vi "Power Spectrum.vi"   [LabVIEW 2024, in "NI_AALPro.lvlib"]
doc: "<p>Computes the <strong>Power Spectrum</strong>, Sxx, of the input sequence <strong>X</strong>. Wire data to the <strong>X</strong> input to determine the polymorphic instance to use or <a href=\"nihelplauncher://docs/csh?context=lvcore_lvhowto_selectingdefaultinstpolyvi\">manually select</a> the instance.\n</p>"
uses:
  NI_AALPro.lvlib
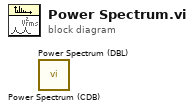
[diagram p0: block diagram]
diagram:
  n1 = call "Power Spectrum (CDB).vi"() -> ()  [unwired: 1 in, 2 out]
  n2 = call "Power Spectrum (DBL).vi"() -> ()  [unwired: 1 in, 2 out]
